vi "RevertorOnNibataserver.vi"() -> ()   [LabVIEW 2013]
uses:
  <vilib>/Utility/config.llb/Read Key (String).vi
  <vilib>/Utility/config.llb/NI_LVConfig.lvlib
panel:
  out "stderr 2":string
  out "stderr":string
  out "concatenated string":string
  in  "Password":string="labview==="
  in  "Username":string="lvadmin"
  in  "Host":string="in-ban-esxi02"
  out "VmPath":string
  in  "Array":bool[](array[boolean])
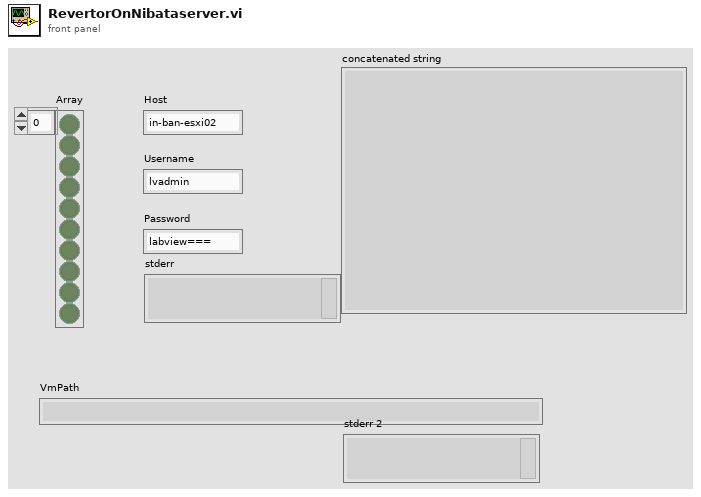
[diagram p1: front panel]
types:
  T1 = typedef "NI_LVConfig.lvlib/Config Data RefNum.ctl" = refnum<k1>
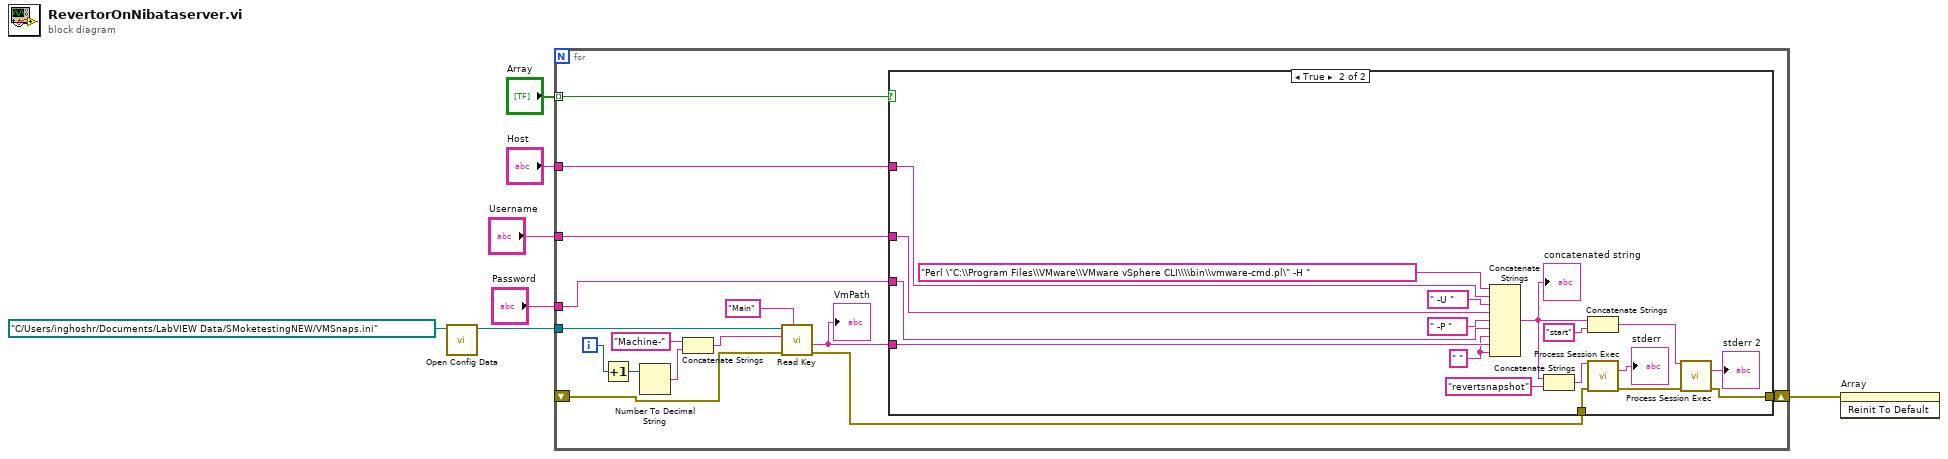
[diagram p0: block diagram]
diagram:
  n1 = call <vilib>:"Open Config Data.vi"("configuration file path"=path "C:/Users/inghoshr/Documents/LabVIEW Data/SMoketestingNEW/VMSnaps.ini") -> ("refnum"=w5:T1)  [unwired: 8 in, 2 out]
  n2 = for {
    tunnel: "Array" -> [w15] mode=indexing
    tunnel: w5 -> [w22]
    tunnel: "Host" -> [w14]
    tunnel: "Username" -> [w13]
    tunnel: "Password" -> [w12]
    shift-right: [w10] -> w1
    shift-left: _ -> [w8]
    i -> [w16]
    n3 = Increment(x=w16) -> (x+1=w17:i32)
    n4 = Number To Decimal String(number=w17) -> (decimal integer string=w20:string)  [unwired: 1 in]
    n5 = Concatenate Strings("Machine-" ("string"), w20) -> (w19:string)
    n6 = call-poly <vilib>:"Read Key.vi"("section"="Main", "error in (no error)"=w8, "key"=w19, "refnum"=w22) -> ("error out"=w9:errorcluster, "value"=w11:string)  [unwired: 4 in, 2 out]
    "VmPath" <- w11
    n7 = case shown="True" w15 {
      tunnel: w14 -> [_ w40]
      tunnel: w13 -> [_ w37]
      tunnel: w12 -> [_ w35]
      tunnel: w11 -> [_ w34]
      tunnel: [_ w24] -> w10
      tunnel: w9 -> [_ w23]
      frame False {
      }
      frame True {
        w33 = " " ("string")
        n8 = Concatenate Strings("Perl \"C:\\Program Files\\VMware\\VMware vSphere CLI\\\\bin\\vmware-cmd.pl\" -H " ("string"), w40, " -U " ("string"), w37, " -P " ("string"), w35, w33, w34, w33) -> (w30:string)
        "concatenated string" <- w30
        n9 = Concatenate Strings(w30, "revertsnapshot" ("string")) -> (w32:string)
        n10 = Concatenate Strings(w30, "start" ("string")) -> (w28:string)
        n11 = call "Process Session Exec.vi"("command line"=w32, "error in (no error)"=w23) -> ("stderr"=→"stderr":string, "error out"=w27:errorcluster)  [unwired: 9 in, 3 out]
        n12 = call "Process Session Exec.vi"("command line"=w28, "error in (no error)"=w27) -> ("stderr"=→"stderr 2":string, "error out"=w24:errorcluster)  [unwired: 9 in, 3 out]
      }
    }
  }
  n13 = invoke on="Array" class="Arr (strict)" method="Reinit To Default"(error in=w1) -> ()  [unwired: 2 in, 3 out]
